vi "Sequential Logic.vi"() -> ()   [LabVIEW 2015]
uses:
  <vilib>/MakerHub/LINX/Private/Type Defs/User Platform.ctl
  <vilib>/MakerHub/LINX/LMH-LINX.lvlib
panel:
  in  "Exit":bool
  out "LS4":bool
  out "LS3":bool
  out "LS2":bool
  out "LS1":bool
  out "C1 Ret":bool
  out "C2 Ret":bool
  out "C2 Ext":bool
  out "C1 Ext":bool
  out "Idle":bool
  in  "Emergency":bool
  in  "Start":bool
  in  "Connect":bool
  in  "Port":refnum<visa-resource-name>
  # "MTE 504 Mechatronics II"
  # "Sequential Logic Control Module"
  # "Arduino PORT"
  # "Current State"
  # "Control Panel"
  # "Transition Condition"
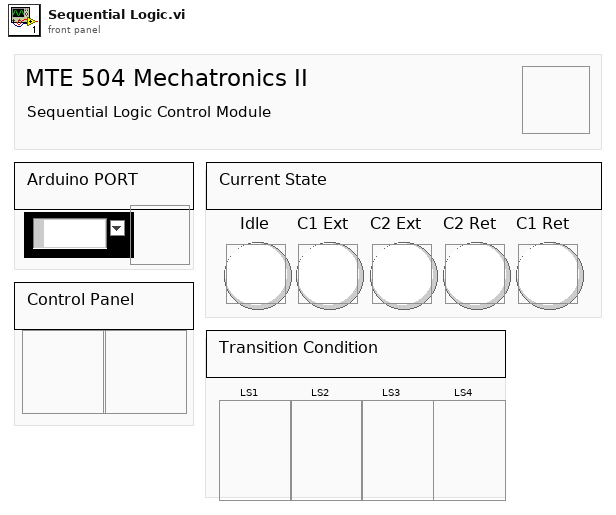
[diagram p1: front panel]
types:
  T1 = typedef "LMH-LINX.lvlib/User Platform.ctl" = enum16{"Default", "LINX", "myRIO"}
  T2 = typedef "LMH-LINX.lvlib/LINX Ref.ctl" = cluster{"Platform":T3, "Interface":T4, "LINX Device Config":T5}
  T3 = typedef "LMH-LINX.lvlib/Platform.ctl" = enum16{"LINX", "myRIO"}
  T4 = typedef "LMH-LINX.lvlib/Interface.ctl" = enum16{"Serial", "TCP"}
  T5 = typedef "LMH-LINX.lvlib/Device.lvlib/LINX Device Config.ctl" = cluster{"Interface":T4, "COM Port":refnum<visa-resource-name>, "TCP Configuration":T6, "Device Family":u8, "Device ID":u8, "Device Name":string, "TCP Ref":refnum<k5>, "Channels":T7}
  T6 = typedef "LMH-LINX.lvlib/Device.lvlib/TCP Config.ctl" = cluster{"IP Address":string, "Port":u16}
  T7 = typedef "LMH-LINX.lvlib/Channels.ctl" = cluster{"DI":u8[], "DO":u8[], "AI":u8[], "AO":u8[], "PWM":u8[], "QE":u8[], "UART":u8[], "I2C 2":u8[], "SPI":u8[], "CAN":u8[], "Servo":u8[], "AI Ref (V)":dbl, "AO Ref (V)":dbl, "AO Resolution (Bits)":u8}
  T8 = enum16{"Idle", "C1 Ext", "C2 Ext", "C2 Ret", "C1 Ret", "Emergency"}
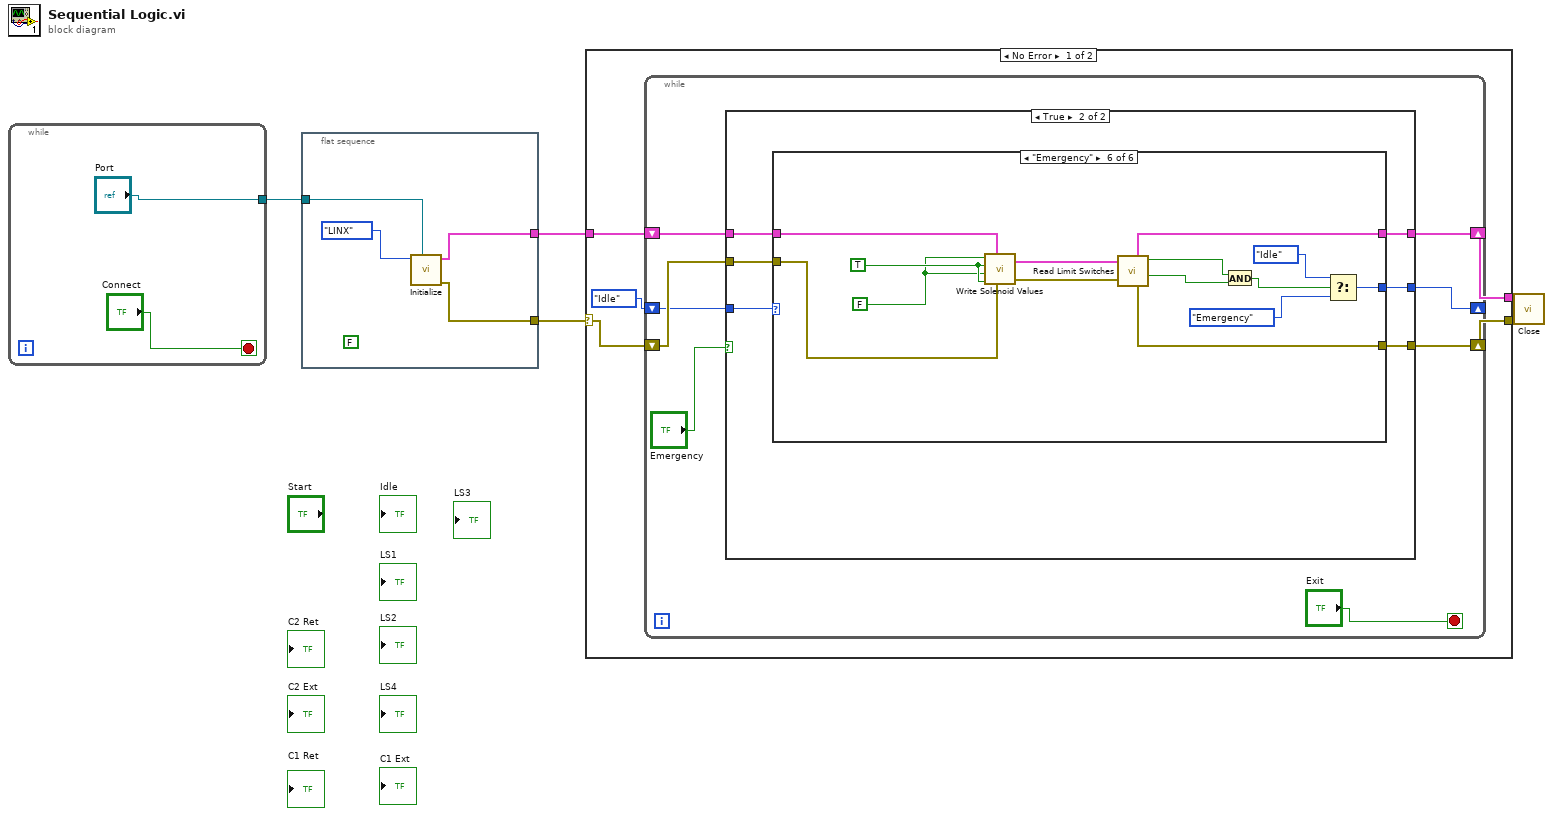
[diagram p0: block diagram]
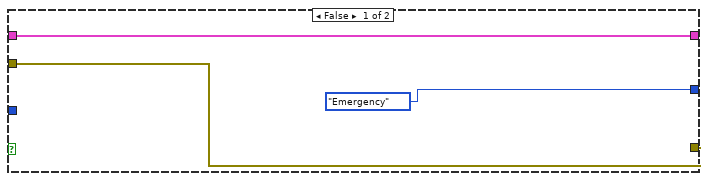
[diagram p2: hidden frame]
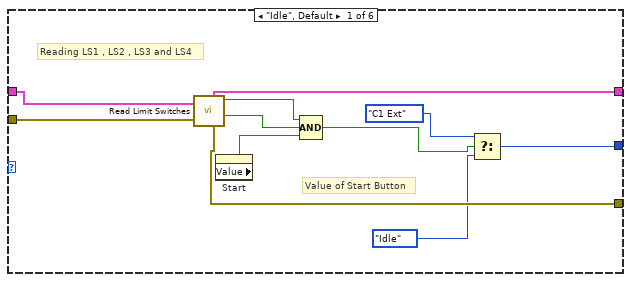
[diagram p3: hidden frame]
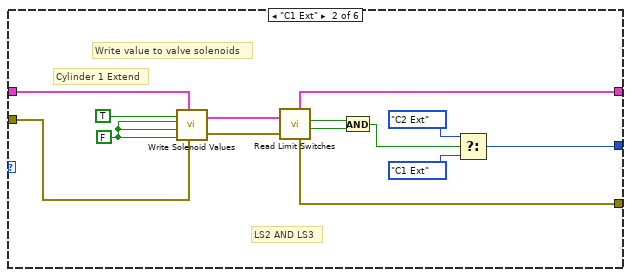
[diagram p4: hidden frame]
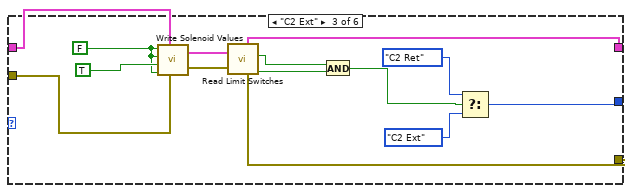
[diagram p5: hidden frame]
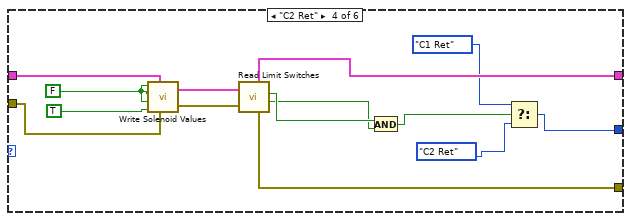
[diagram p6: hidden frame]
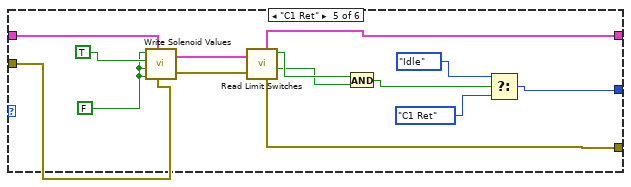
[diagram p7: hidden frame]
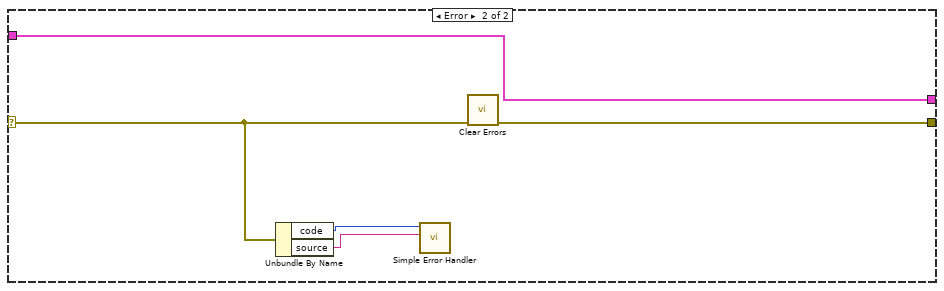
[diagram p8: hidden frame]
diagram:
  n1 = while {
    tunnel: ["Port"] -> w5
    stop <- "Connect" stop-if-true
  }
  n2 = flat-sequence {
    tunnel: w5 -> [w11]
    tunnel: [w9] -> w4
    tunnel: [w8] -> w3
    frame #0 {
      (unwired) FALSE ("Visible")
      n3 = call <vilib>:"Initialize.vi"("Serial Port"=w11, "Platform"=User_Platform."LINX") -> ("Error Out"=w9:errorcluster, "LINX Ref"=w8:T2)  [unwired: 7 in, 1 out]
    }
  }
  n4 = case shown="No Error" w4 {
    selector: w4 -> [w15 w118]
    tunnel: [w13 w119] -> w1
    tunnel: w3 -> [w16 w115]
    tunnel: [w14 w115] -> w2
    frame No Error {
      n5 = while {
        shift-right: [w22] -> w14
        shift-left: w16 -> [w24]
        shift-right: [w21] -> w13
        shift-left: w15 -> [w23]
        shift-right: [w20] -> _
        shift-left: T8."Idle" -> [w19]
        stop <- "Exit" stop-if-true
        n6 = case shown="True" "Emergency" {
          tunnel: w24 -> [w26 w33]
          tunnel: w23 -> [w25 w32]
          tunnel: [w26 w31] -> w22
          tunnel: [w25 w30] -> w21
          tunnel: [T8."Emergency" w29] -> w20
          tunnel: w19 -> [_ w28]
          frame False {
          }
          frame True {
            n7 = case shown="\"Emergency\"" w28 {
              tunnel: w33 -> [w44 w58 w72 w86 w100 w114]
              tunnel: w32 -> [w43 w57 w71 w85 w99 w113]
              tunnel: [w39 w52 w67 w82 w94 w108] -> w31
              tunnel: [w38 w51 w66 w81 w93 w107] -> w30
              tunnel: [w36 w47 w62 w79 w89 w101] -> w29
              frame "Idle", Default {
                # "Value of Start Button"
                # "Reading LS1 , LS2 , LS3 and LS4"
                n8 = call "Read Limit Switches.vi"("LINX Resource"=w44, "Error In"=w43) -> ("LINX Resource 2"=w39:T2, "Error Out"=w38:errorcluster, "LS1"=w42:bool, "LS3"=w41:bool)  [unwired: 2 out]
                n9 = property on="Start" class="Bool (strict)"() -> ("Value"=w40:bool)  [unwired: 2 in, 2 out]
                n10 = Compound Arithmetic op=AND(w42, w41, w40) -> (w37:bool)
                n11 = Select(t=T8."C1 Ext", s=w37, f=T8."Idle") -> (s? t:f=w36:T8)
              }
              frame "C1 Ext" {
                w55 = FALSE
                # "LS2 AND LS3"
                # "Cylinder 1 Extend"
                # "Write value to valve solenoids"
                n12 = call "Write Solenoid Values.vi"("Error In"=w57, "LINX Resource"=w58, "C2 Ret Value"=w55, "C2 Ext Value"=w55, "C1 Ret Value"=w55, "C1 Ext Value"=TRUE) -> ("Error Out"=w53:errorcluster, "LINX Resource 2"=w54:T2)
                n13 = call "Read Limit Switches.vi"("LINX Resource"=w54, "Error In"=w53) -> ("LINX Resource 2"=w52:T2, "Error Out"=w51:errorcluster, "LS2"=w50:bool, "LS3"=w49:bool)  [unwired: 2 out]
                n14 = And(x=w50, y=w49) -> (x .and. y?=w48:bool)
                n15 = Select(t=T8."C2 Ext", s=w48, f=T8."C1 Ext") -> (s? t:f=w47:T8)
              }
              frame "C2 Ext" {
                w61 = FALSE
                n16 = call "Write Solenoid Values.vi"("Error In"=w71, "LINX Resource"=w72, "C2 Ret Value"=w61, "C2 Ext Value"=TRUE, "C1 Ret Value"=w61, "C1 Ext Value"=w61) -> ("Error Out"=w68:errorcluster, "LINX Resource 2"=w69:T2)
                n17 = call "Read Limit Switches.vi"("LINX Resource"=w69, "Error In"=w68) -> ("LINX Resource 2"=w67:T2, "Error Out"=w66:errorcluster, "LS2"=w65:bool, "LS4"=w64:bool)  [unwired: 2 out]
                n18 = And(x=w65, y=w64) -> (x .and. y?=w63:bool)
                n19 = Select(t=T8."C2 Ret", s=w63, f=T8."C2 Ext") -> (s? t:f=w62:T8)
              }
              frame "C2 Ret" {
                w75 = FALSE
                n20 = call "Write Solenoid Values.vi"("Error In"=w85, "LINX Resource"=w86, "C2 Ret Value"=TRUE, "C2 Ext Value"=w75, "C1 Ret Value"=w75, "C1 Ext Value"=w75) -> ("Error Out"=w83:errorcluster, "LINX Resource 2"=w84:T2)
                n21 = call "Read Limit Switches.vi"("LINX Resource"=w84, "Error In"=w83) -> ("LINX Resource 2"=w82:T2, "Error Out"=w81:errorcluster, "LS2"=w78:bool, "LS3"=w77:bool)  [unwired: 2 out]
                n22 = And(x=w78, y=w77) -> (x .and. y?=w80:bool)
                n23 = Select(t=T8."C1 Ret", s=w80, f=T8."C2 Ret") -> (s? t:f=w79:T8)
              }
              frame "C1 Ret" {
                w97 = FALSE
                n24 = call "Write Solenoid Values.vi"("Error In"=w99, "LINX Resource"=w100, "C2 Ret Value"=w97, "C2 Ext Value"=w97, "C1 Ret Value"=TRUE, "C1 Ext Value"=w97) -> ("Error Out"=w95:errorcluster, "LINX Resource 2"=w96:T2)
                n25 = call "Read Limit Switches.vi"("LINX Resource"=w96, "Error In"=w95) -> ("LINX Resource 2"=w94:T2, "Error Out"=w93:errorcluster, "LS1"=w92:bool, "LS3"=w91:bool)  [unwired: 2 out]
                n26 = And(x=w92, y=w91) -> (x .and. y?=w90:bool)
                n27 = Select(t=T8."Idle", s=w90, f=T8."C1 Ret") -> (s? t:f=w89:T8)
              }
              frame "Emergency" {
                w109 = FALSE
                w110 = TRUE
                n28 = call "Write Solenoid Values.vi"("Error In"=w113, "LINX Resource"=w114, "C2 Ret Value"=w110, "C2 Ext Value"=w109, "C1 Ret Value"=w110, "C1 Ext Value"=w109) -> ("Error Out"=w111:errorcluster, "LINX Resource 2"=w112:T2)
                n29 = call "Read Limit Switches.vi"("LINX Resource"=w112, "Error In"=w111) -> ("LINX Resource 2"=w108:T2, "Error Out"=w107:errorcluster, "LS1"=w106:bool, "LS3"=w105:bool)  [unwired: 2 out]
                n30 = And(x=w106, y=w105) -> (x .and. y?=w104:bool)
                n31 = Select(t=T8."Idle", s=w104, f=T8."Emergency") -> (s? t:f=w101:T8)
              }
            }
          }
        }
      }
    }
    frame Error {
      n32 = Unbundle By Name(w118) -> ("code"=w117:i32, "source"=w116:string)
      n33 = call <vilib>:"Simple Error Handler.vi"("error code (no error:0)"=w117, "error source (\" \")"=w116) -> ()  [unwired: 3 in, 5 out]
      n34 = call <vilib>:"Clear Errors.vi"("error in (no error)"=w118) -> ("error out"=w119:errorcluster)  [unwired: 5 in, 1 out]
    }
  }
  n35 = call <vilib>:"Close.vi"("Error In"=w1, "LINX Resource"=w2) -> ()  [unwired: 8 in, 2 out]
